vi "CreateInmatrix.vi"() -> ()   [LabVIEW 2014]
uses:
  <vilib>/Analysis/Matrix/Datatypes/RealMatrix.ctl
  <vilib>/Utility/file.llb/Read From Spreadsheet File (DBL).vi
  <vilib>/Analysis/Matrix/NI_Matrix.lvlib
panel:
  out "LDA_matrix":T1
  out "in":dbl[](array[numeric])
  in  "ERP Non-Target":path caption="ERP_Nontarget"
  in  "ERP Target":path caption="ERP_Target"
  in  "penter":dbl=0.01
  in  "premove":dbl=0.1
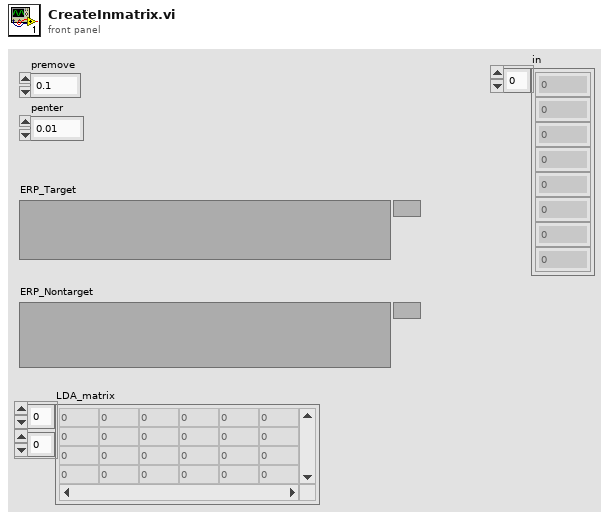
[diagram p1: front panel]
types:
  T1 = typedef "NI_Matrix.lvlib/RealMatrix.ctl" = dbl[][]
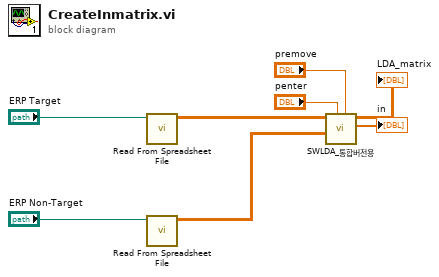
[diagram p0: block diagram]
diagram:
  n1 = call-poly <vilib>:"Read From Spreadsheet File.vi"("file path (dialog if empty)"="ERP Target") -> ("all rows"=w5:dbl[][])  [unwired: 6 in, 4 out]
  n2 = call-poly <vilib>:"Read From Spreadsheet File.vi"("file path (dialog if empty)"="ERP Non-Target") -> ("all rows"=w3:dbl[][])  [unwired: 6 in, 4 out]
  n3 = call "SWLDA_통합버전용.vi"("premove"="premove", "penter"="penter", "ERP_Nontarget"=w3, "ERP_Target"=w5) -> ("in"=→"in":dbl[], "LDA_matrix"=→"LDA_matrix":T1)  [unwired: 5 in, 1 out]
